vi "FEA_Model_LEMP_Caller.vi"(8 "error in (no error)":errorcluster, 10 "Node of interest":i32, 11 "FEA_Model in":refnum<class "FEA_Model.lvclass">) -> (0 "error out":errorcluster, 2 "Frequency":dbl, 3 "FEA_Model out":refnum<class "FEA_Model.lvclass">)   [LabVIEW 2021, in "FEA_Model.lvclass"]
uses:
  FEA_Model.lvclass
  FEA_Model.lvclass/FEA_Model.ctl
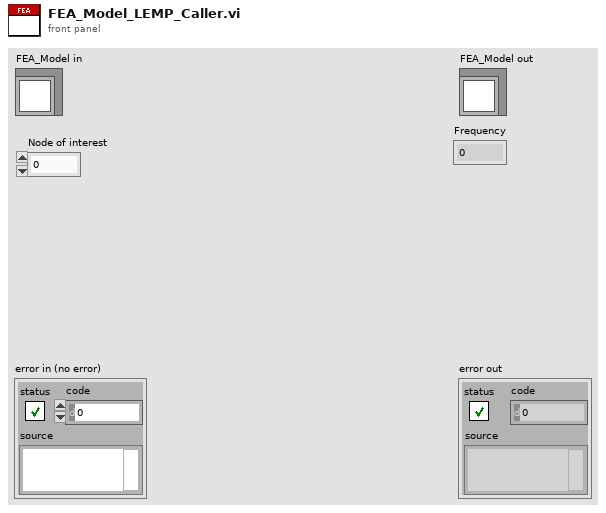
[diagram p1: front panel]
types:
  T1 = cluster{"Eigenvalues":dbl[], "SquareT Eigenvectors":dbl[][], "1/deltaStiff":dbl}
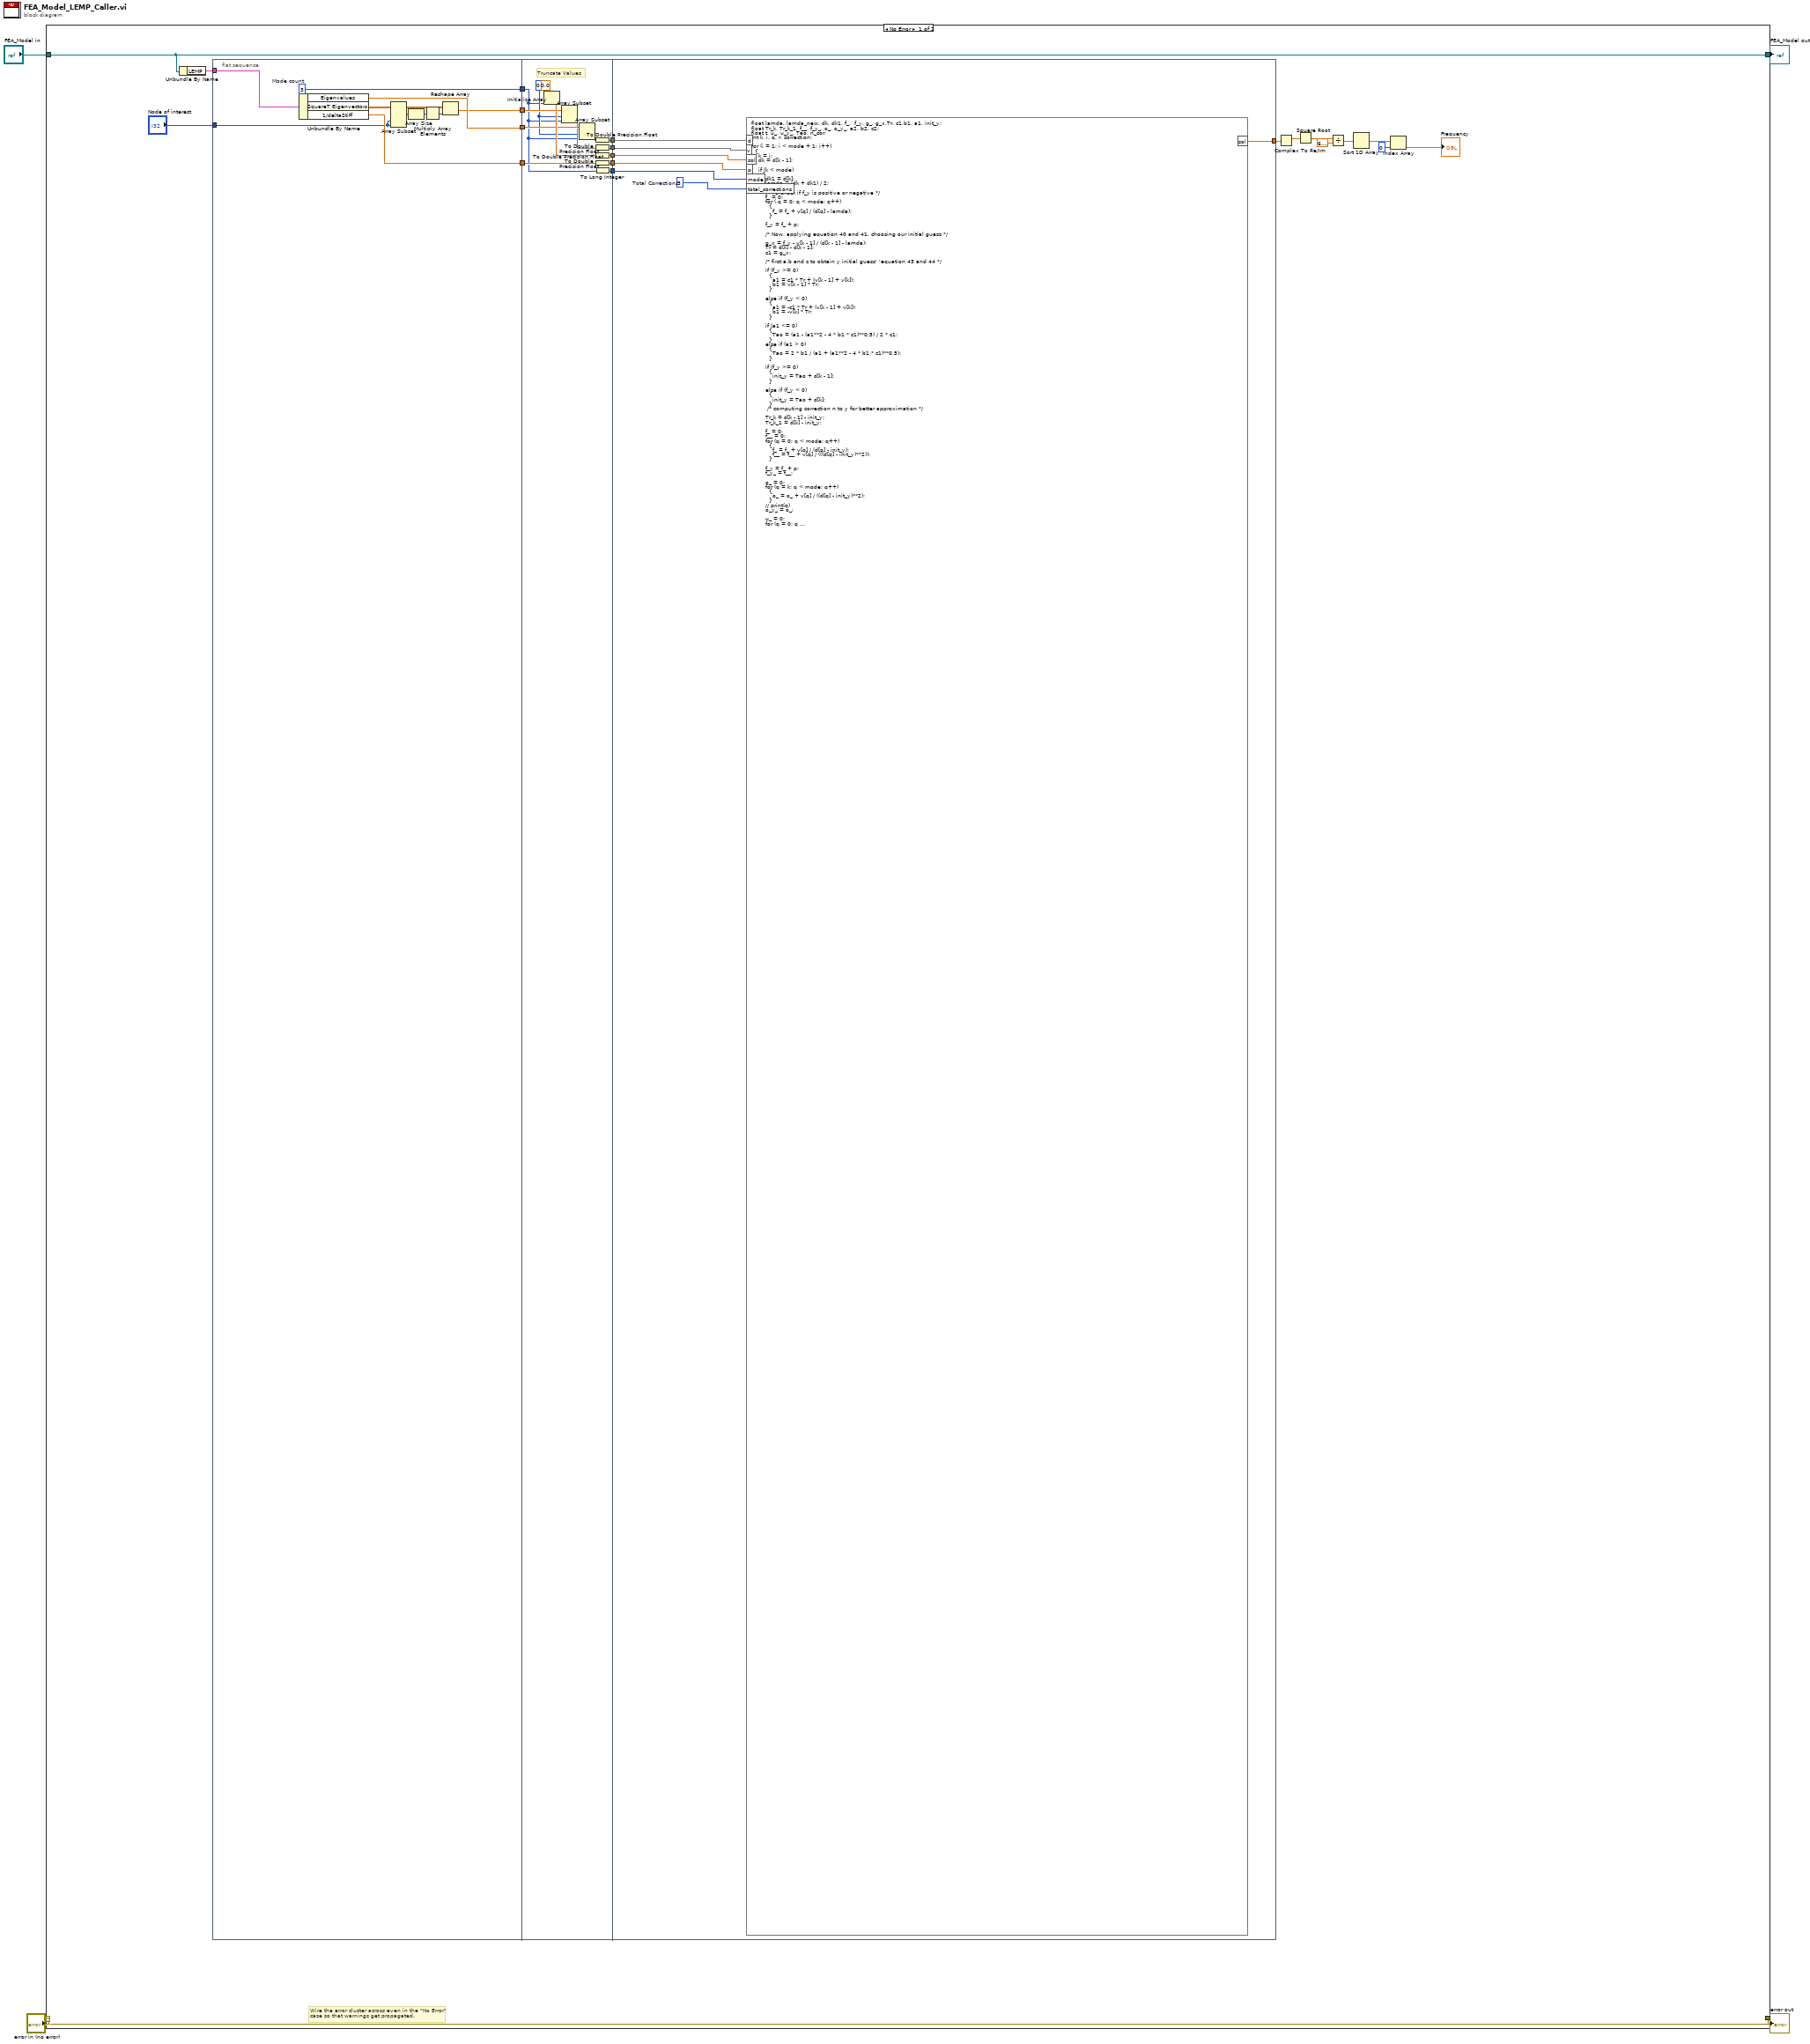
[diagram p0: block diagram]
diagram:
  n1 = case shown="No Error" "error in (no error)" {
    selector: "error in (no error)" -> [w25 w58]
    tunnel: [w25 w58] -> w3
    tunnel: "FEA_Model in" -> [w7 w57]
    tunnel: [w7 w57] -> w1
    frame No Error {
      # "Wire the error cluster across even in the \"No Error\"\ncase so that warnings get propagated."
      n2 = Unbundle By Name(w7) -> ("LEMP"=w24:T1)
      n3 = flat-sequence {
        tunnel: [w29] -> w23
        tunnel: [w31] -> w22
        tunnel: [w30] -> w21
        tunnel: [w28] -> w20
        tunnel: "Node of interest" -> [w27]
        tunnel: w24 -> [w26]
        tunnel: [w41] -> w19
        tunnel: [w39] -> w18
        tunnel: [w37] -> w16
        tunnel: [w38] -> w15
        tunnel: [w36] -> w17
        tunnel: w23 -> [w46]
        tunnel: w22 -> [w45]
        tunnel: w21 -> [w49]
        tunnel: w20 -> [w40]
        tunnel: w19 -> [w56]
        tunnel: w18 -> [w55]
        tunnel: w17 -> [w52]
        tunnel: w16 -> [w53]
        tunnel: w15 -> [w54]
        tunnel: [w51] -> w8
        frame #0 {
          w28 = 3  # Mode count
          n4 = Unbundle By Name(w26) -> ("Eigenvalues"=w31:dbl[], "SquareT Eigenvectors"=w35:dbl[][], "1/deltaStiff"=w30:dbl)
          n5 = Array Subset(array=w35, index (col)=w27, length (col)=w27) -> (w34:dbl[][])  [unwired: 2 in]
          n6 = Array Size(array=w34) -> (size(s)=w32:i32[])
          n7 = Multiply Array Elements(1:w32) -> (0:w33:i32)
          n8 = Reshape Array(w34, w33) -> (w29:dbl[])
        }
        frame #1 {
          w43 = 0
          # "Truncate Values"
          n9 = Initialize Array(0.0, w40) -> (w47:dbl[])
          n10 = Array Subset(array=w46, index=w43, length=w40) -> (w44:dbl[])
          n11 = Array Subset(array=w45, index=w43, length=w40) -> (w42:dbl[])
          n12 = To Double Precision Float(number=w42) -> (double precision float=w41:dbl[])
          n13 = To Double Precision Float(number=w44) -> (double precision float=w39:dbl[])
          n14 = To Double Precision Float(number=w47) -> (double precision float=w38:dbl[])
          n15 = To Double Precision Float(number=w49) -> (double precision float=w37:dbl)
          n16 = To Long Integer(number=w40) -> (32bit integer=w36:i32)
        }
        frame #2 {
          w50 = 3  # Total Corrections
          n17 = formula code="float lamda, lamda_new, dk, dk1, f_,  f_y, g_, g_x,Tr, c1,b1, a1, init_y;\nfloat Tr_k, Tr_k_1, f__, f_y_, o_, o_y_, a2, b2, c2;\nfloat t, u_, u_y_, Tao, n_cor;\nint k, i, q, r, correction;\n\nfor (i = 1; i < mode + 1; i++)\n  {\n    k = i;\n    dk = d[k - 1];\n\n    if (k < mode)\n      {\n        dk1 = d[k];\n        lamda = (dk + dk1) / 2;\n\n        /* To check if f_y is positive or negative */\n        f_ = 0;\n        for ( q = 0; q < mode; q++)\n          {\n            f_ = f_ + v[q] / (d[q] - lamda);\n          }\n\n        f_y = f_ + p;\n\n        /* Now, applying equation 40 and 41, choosing our initial guess */\n\n        g_x = f_y - v[k - 1] / (d[k - 1] - lamda);\n        Tr = d[k] - d[k - 1];\n        c1 = g_x;\n\n        /* first a,b and c to obtain y initial guess' 'equation 43 and 44 */\n\n        if (f_y >= 0)\n          {\n            a1 = c1 * Tr + (v[k - 1] + v[k]);\n            b1 = v[k - 1] * Tr;\n          }\n\n        else if (f_y < 0)\n          {\n            a1 = -c1 * Tr + (v[k - 1] + v[k]);\n            b1 = -v[k] * Tr;\n          }\n\n        if (a1 <= 0)\n          {\n            Tao = (a1 - (a1**2 - 4 * b1 * c1)**0.5) / 2 * c1;\n          }\n        else if (a1 > 0)\n          {\n            Tao = 2 * b1 / (a1 + (a1**2 - 4 * b1 * c1)**0.5);\n          }\n\n        if (f_y >= 0)\n          {\n            init_y = Tao + d[k - 1];\n          }\n\n        else if (f_y < 0)\n          {\n            init_y = Tao + d[k];\n          }\n         /* computing correction n to y for better approximation */\n\n        Tr_k = d[k - 1] - init_y;\n        Tr_k_1 = d[k] - init_y;\n\n        f_ = 0;\n        f__ = 0;\n        for (q = 0; q < mode; q++)\n          {\n            f_ = f_ + v[q] / (d[q] - init_y);\n            f__ = f__ + v[q] / (((d[q] - init_y)**2));\n          }\n\n        f_y = f_ + p;\n        f_y_ = f__;\n\n        o_ = 0;\n        for (q = k; q < mode; q++)\n          {\n            o_ = o_ + v[q] / ((d[q] - init_y)**2);\n          }\n        // print(q)\n        o_y_ = o_;\n\n        u_ = 0;\n        for (q = 0; q < mode; q++)\n          {\n            u_ = u_ + v[q] / ((d[q] - init_y)**2);\n          }\n        // print(q)\n\n        u_y_ = u_;\n        /*'second a, b and c for final correction' */\n\n        a2 = (Tr_k + Tr_k_1) * f_y - Tr_k * Tr_k_1 * f_y_;\n        b2 = Tr_k * Tr_k_1 * f_y;\n\n        if (f_y >= 0)\n          {\n            c2 = f_y - Tr_k_1 * f_y_ - u_y_ * (d[k - 1] - d[k]);\n          }\n\n        else if (f_y < 0)\n          {\n            c2 = f_y - Tr_k * f_y_ - o_y_ * (d[k] - d[k - 1]);\n          }\n\n        if (a2 <= 0)\n          {\n            n_cor = (a2 - (a2**2 - 4 * b2 * c2)**0.5) / 2 * c2;\n          }\n\n        else if (a2 > 0)\n          {\n            n_cor = 2 * b2 / (a2 + (a2**2 - 4 * b2 * c2)**0.5);\n          }\n\n        lamda_new = init_y + n_cor;\n        /*computing second correction n to y for better approximation */\n        // init_y = lamda_new;\n\n        sol[k - 1] = lamda_new;\n      }\n\n    else if (k == mode)\n      {\n        t = 0;\n        for (r = 0; r < mode; r++)\n          {\n            t = t + (v[r]**2);\n          }\n\n        float d6;\n\n        d6 = d[k - 1] + t / p;\n\n        lamda = (d6 + d[k - 1]) / 2;\n\n        //'To check if f_y is positive or negative'\n\n        f_ = 0;\n        for( q = 0; q < mode; q++)\n          {\n            f_ = f_ + v[q] / (d[q] - lamda);\n          }\n\n        f_y = f_ + p;\n\n        //'Now, applying equation 40 and 41, choosing our initial guess'\n        /*g_ = 0;\n           for( q = 0; q<n; q++)\n           {\n           g_ = g_ + v[q]/(d[q]-lamda);\n           }\n\n           g_x = g_ + p; */\n\n        g_x = f_y - v[k - 1] / (d[k - 1] - lamda);\n        Tr = d[k - 1] - d[k - 2];\n        c1 = g_x;\n\n        //'first a,b and c to obtain y initial guess' 'equation 43 and 44'\n        if (f_y <= 0)\n          {\n            a1 = c1 * Tr + (v[k - 2] + v[k - 1]);\n            b1 = v[k - 1] * Tr;\n          }\n\n        else if (f_y > 0)\n          {\n            a1 = -c1 * Tr + (v[k - 2] + v[k - 1]);\n            b1 = -v[k - 1] * Tr;\n          }\n\n        if (a1 <= 0)\n          {\n            Tao = (a1 + (a1**2 - 4 * b1 * c1)**0.5) / 2 * c1;\n          }\n\n        else if (a1 > 0)\n          {\n            Tao = 2 * b1 / (a1 - (a1**2 - 4 * b1 * c1)**0.5);\n          }\n\n        init_y = Tao + d[k - 1];\n\n        //'computing correction n to y for better approximation'\n        for (correction = 1; correction < total_corrections; correction++)\n          {\n\n            Tr_k = d[k - 1] - init_y;\n            Tr_k_1 = d6 - init_y;\n\n            f_ = 0;\n            f__ = 0;\n            for (q = 0; q < mode; q++)\n              {\n                f_ = f_ + v[q] / (d[q] - init_y);\n                f__ = f__ + v[q] / ((d[q] - init_y)**2);\n              }\n\n            f_y = f_ + p;\n            f_y_ = f__;\n\n            u_ = 0;\n            for (q = 0; q < mode; q++)\n              {\n                u_ = u_ + v[q] / ((d[q] - init_y)**2);\n              }\n\n            u_y_ = u_;\n            //'second a, b and c for final correction'\n\n            a2 = (Tr_k + Tr_k_1) * f_y - Tr_k * Tr_k_1 * f_y_;\n            b2 = Tr_k * Tr_k_1 * f_y;\n            c2 = f_y - Tr_k * u_y_ - (v[k - 1] / Tr_k_1);\n\n            if (a2 <= 0)\n              {\n                n_cor = (a2 - (a2**2 - 4 * b2 * c2)**0.5) / 2 * c2;\n              }\n\n            else if (a2 > 0)\n              {\n                n_cor = 2 * b2 / (a2 + (a2**2 - 4 * b2 * c2)**0.5);\n              }\n\n            lamda_new = init_y + n_cor;\n            init_y = lamda_new;\n          }\n        sol[mode - 1] = lamda_new;\n      }\n  }"("d"=w56, "v"=w55, "p"=w53, "mode"=w52, "sol"=w54, "total_corrections"=w50) -> ("sol"=w51:dbl[])
        }
      }
      n18 = Complex To Re/Im ("Complex To Cartesian.vi")(x + iy=w8) -> (x=w14:dbl[])  [unwired: 1 out]
      n19 = Square Root ("Square Root.vi")(x=w14) -> (sqrt(x)=w13:dbl[])
      n20 = Divide(x=w13, y=6.283185307179586) -> (x/y=w9:dbl[])
      n21 = Sort 1D Array(array=w9) -> (sorted array=w11:dbl[])
      n22 = Index Array(array=w11, index=0) -> (element=→"Frequency":dbl)
    }
    frame Error {
    }
  }
  "error out" <- w3
  "FEA_Model out" <- w1
